vi "numero_imagens.vi"() -> ()   [LabVIEW 2016]
panel:
  in  "Número de Imagens":dbl
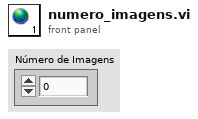
[diagram p1: front panel]
diagram:
